vi "Initialize Diagnostics Main.vi"(8 "error in (no error)":errorcluster, 10 "This VI":refnum<vi>, 11 "Parameters":T1={"Properties"={"Name"="", "CAN"={"Database File"=path "", "CAN Interface"=enum."CAN0", "Baud Rate"=0, "Diagnostic Protocol"=enum."GMLAN", "Transport Protocol"=enum."ISO TP - Normal Mode", "Transmit ID"=0, "Receive ID"=0, "Transmit Extension"=0, "Receive Extension"=0, "Receive UUDT ID"=0, "Enable Stream"=TRUE, "VW TP Channel ID"=0, "Security"={"Source DLL Path"=path "", "Security Level"=1, "Target DLL Path"=path ""}, "Fill Frame"=FALSE, "Fill Byte"=255, "Termination"=FALSE}, "FPGA Settings"={"RT Bitfile Path"=path "", "RIO Device"=0, "Enable"=FALSE}, "PIDs"=[], "PID Lookup"=variant, "CPIDs"=[], "CPID Lookup"=variant, "DIDs"=[], "DID Lookup"=variant, "DPIDs"=[], "DPID Lookup"=variant, "DTC descriptor"={"DTC Byte Length"=2, "Status Byte Length"=1, "Add Data Byte Length"=1, "Byte Order"=enum."Motorola"}, "Routine.Start.Cmd Lookup"=variant, "Routine.Status.Cmd Lookup"=variant, "Routine.Stop.Cmd Lookup"=variant, "IO.Cmd Lookup"=variant, "IO.Resp Lookup"=variant, "Routine.Start.Resp Lookup"=variant, "Routine.Status.Resp Lookup"=variant, "Routine.Stop.Resp Lookup"=variant, "Memory.Write Lookup"=variant, "Memory.Read Lookup"=variant}, "ChanRefs"={"ToVS.PIDs"={"Name"="", "Write to VS Engine FIFO"=refnum, "Pairs"={"Refs"=[], "Values"=[]}}, "ToVS.DIDs"={"Name"="", "Write to VS Engine FIFO"=refnum, "Pairs"={"Refs"=[], "Values"=[]}}, "ToVS.DTCs"={"Name"="", "Write to VS Engine FIFO"=refnum, "Pairs"={"Refs"=[], "Values"=[]}}, "ToVS.DTCCount"={"Name"="", "Write to VS Engine FIFO"=refnum, "Pairs"={"Refs"=[], "Values"=[]}}, "ToVS.Status"={"Name"="", "Write to VS Engine FIFO"=refnum, "Pairs"={"Refs"=[], "Values"=[]}}, "FromVS.CPIDs"={"Name"="", "Read from VS Engine FIFO"=refnum, "Pairs"={"Refs"=[], "Values"=[]}}, "Cmds"={"Name"="", "Write to VS Engine FIFO"=refnum, "Read from VS Engine FIFO"=refnum, "Pairs"={"Chan Refs"=[], "Prev. Values"=[]}}, "ToVS.Routine.Start"={"Name"="", "Write to VS Engine FIFO"=refnum, "Pairs"={"Refs"=[], "Values"=[]}}, "FromVS.Routine.Start"={"Name"="", "Read from VS Engine FIFO"=refnum, "Pairs"={"Refs"=[], "Values"=[]}}, "ToVS.Routine.Stop"={"Name"="", "Write to VS Engine FIFO"=refnum, "Pairs"={"Refs"=[], "Values"=[]}}, "FromVS.Routine.Stop"={"Name"="", "Read from VS Engine FIFO"=refnum, "Pairs"={"Refs"=[], "Values"=[]}}, "ToVS.Routine.Status"={"Name"="", "Write to VS Engine FIFO"=refnum, "Pairs"={"Refs"=[], "Values"=[]}}, "FromVS.Routine.Status"={"Name"="", "Read from VS Engine FIFO"=refnum, "Pairs"={"Refs"=[], "Values"=[]}}, "FromVS.IO.Cmd"={"Name"="", "Read from VS Engine FIFO"=refnum, "Pairs"={"Refs"=[], "Values"=[]}}, "ToVS.IO.Resp"={"Name"="", "Write to VS Engine FIFO"=refnum, "Pairs"={"Refs"=[], "Values"=[]}}, "FromVS.WriteMemory"={"Name"="", "Read from VS Engine FIFO"=refnum, "Pairs"={"Refs"=[], "Values"=[]}}, "ToVS.ReadMemory"={"Name"="", "Write to VS Engine FIFO"=refnum, "Pairs"={"Refs"=[], "Values"=[]}}}} {"ChanRefs"."ToVS.ReadMemory"."Pairs"."Refs" format="%.0x"; "ChanRefs"."FromVS.WriteMemory"."Pairs"."Refs"."Data Reference" format="%.0x"; "ChanRefs"."ToVS.IO.Resp"."Pairs"."Refs" format="%.0x"; "ChanRefs"."FromVS.IO.Cmd"."Pairs"."Refs"."Data Reference" format="%.0x"; "ChanRefs"."FromVS.Routine.Status"."Pairs"."Refs"."Data Reference" format="%.0x"; "ChanRefs"."ToVS.Routine.Status"."Pairs"."Refs" format="%.0x"; "ChanRefs"."FromVS.Routine.Stop"."Pairs"."Refs"."Data Reference" format="%.0x"; "ChanRefs"."ToVS.Routine.Stop"."Pairs"."Refs" format="%.0x"; "ChanRefs"."FromVS.Routine.Start"."Pairs"."Refs"."Data Reference" format="%.0x"; "ChanRefs"."ToVS.Routine.Start"."Pairs"."Refs" format="%.0x"; "ChanRefs"."Cmds"."Pairs"."Chan Refs" format="%.0x"; "ChanRefs"."FromVS.CPIDs"."Pairs"."Refs"."Data Reference" format="%.0x"; "ChanRefs"."ToVS.Status"."Pairs"."Refs" format="%.0x"; "ChanRefs"."ToVS.DTCCount"."Pairs"."Refs" format="%.0x"; "ChanRefs"."ToVS.DTCs"."Pairs"."Refs" format="%.0x"; "ChanRefs"."ToVS.PIDs"."Pairs"."Refs" format="%.0x"; "ChanRefs"."ToVS.DIDs"."Pairs"."Refs" format="%.0x"; "Properties"."CPIDs"."Signals"."Byte Order" items=["Little Endian", "Big Endian"]; "Properties"."CPIDs"."Signals"."Data Type" items=["Signed", "Unsigned", "IEEE Float"]; "Properties"."DIDs"."Signals"."Byte Order" items=["Little Endian", "Big Endian"]; "Properties"."DIDs"."Signals"."Data Type" items=["Signed", "Unsigned", "IEEE Float"]; "Properties"."CAN"."Fill Byte" format="%.0x"; "Properties"."CAN"."VW TP Channel ID" format="%.0x"; "Properties"."CAN"."Receive UUDT ID" format="%.0x"; "Properties"."CAN"."Receive Extension" format="%.0x"; "Properties"."CAN"."Transmit Extension" format="%.0x"; "Properties"."CAN"."Receive ID" format="%.0x"; "Properties"."CAN"."Transmit ID" format="%.0x"; "Properties"."PIDs"."Signals"."Byte Order" items=["Little Endian", "Big Endian"]; "Properties"."PIDs"."Signals"."Data Type" items=["Signed", "Unsigned", "IEEE Float"]}) -> (0 "error out":errorcluster {"code" min=0 max=0}, 3 "State Variables Out":T20={"TCP Refs"={"Connection List"=refnum, "listener ID"=refnum}, "Stop"=refnum, "Top VI"=refnum, "Parameters"={"Properties"={"Name"="", "CAN"={"Database File"=path "", "CAN Interface"=enum."CAN0", "Baud Rate"=0, "Diagnostic Protocol"=enum."GMLAN", "Transport Protocol"=enum."ISO TP - Normal Mode", "Transmit ID"=0, "Receive ID"=0, "Transmit Extension"=0, "Receive Extension"=0, "Receive UUDT ID"=0, "Enable Stream"=TRUE, "VW TP Channel ID"=0, "Security"={"Source DLL Path"=path "", "Security Level"=1, "Target DLL Path"=path ""}, "Fill Frame"=FALSE, "Fill Byte"=255, "Termination"=FALSE}, "FPGA Settings"={"RT Bitfile Path"=path "", "RIO Device"=0, "Enable"=FALSE}, "PIDs"=[], "PID Lookup"=variant, "CPIDs"=[], "CPID Lookup"=variant, "DIDs"=[], "DID Lookup"=variant, "DPIDs"=[], "DPID Lookup"=variant, "DTC descriptor"={"DTC Byte Length"=2, "Status Byte Length"=1, "Add Data Byte Length"=1, "Byte Order"=enum."Motorola"}, "Routine.Start.Cmd Lookup"=variant, "Routine.Status.Cmd Lookup"=variant, "Routine.Stop.Cmd Lookup"=variant, "IO.Cmd Lookup"=variant, "IO.Resp Lookup"=variant, "Routine.Start.Resp Lookup"=variant, "Routine.Status.Resp Lookup"=variant, "Routine.Stop.Resp Lookup"=variant, "Memory.Write Lookup"=variant, "Memory.Read Lookup"=variant}, "ChanRefs"={"ToVS.PIDs"={"Name"="", "Write to VS Engine FIFO"=refnum, "Pairs"={"Refs"=[], "Values"=[]}}, "ToVS.DIDs"={"Name"="", "Write to VS Engine FIFO"=refnum, "Pairs"={"Refs"=[], "Values"=[]}}, "ToVS.DTCs"={"Name"="", "Write to VS Engine FIFO"=refnum, "Pairs"={"Refs"=[], "Values"=[]}}, "ToVS.DTCCount"={"Name"="", "Write to VS Engine FIFO"=refnum, "Pairs"={"Refs"=[], "Values"=[]}}, "ToVS.Status"={"Name"="", "Write to VS Engine FIFO"=refnum, "Pairs"={"Refs"=[], "Values"=[]}}, "FromVS.CPIDs"={"Name"="", "Read from VS Engine FIFO"=refnum, "Pairs"={"Refs"=[], "Values"=[]}}, "Cmds"={"Name"="", "Write to VS Engine FIFO"=refnum, "Read from VS Engine FIFO"=refnum, "Pairs"={"Chan Refs"=[], "Prev. Values"=[]}}, "ToVS.Routine.Start"={"Name"="", "Write to VS Engine FIFO"=refnum, "Pairs"={"Refs"=[], "Values"=[]}}, "FromVS.Routine.Start"={"Name"="", "Read from VS Engine FIFO"=refnum, "Pairs"={"Refs"=[], "Values"=[]}}, "ToVS.Routine.Stop"={"Name"="", "Write to VS Engine FIFO"=refnum, "Pairs"={"Refs"=[], "Values"=[]}}, "FromVS.Routine.Stop"={"Name"="", "Read from VS Engine FIFO"=refnum, "Pairs"={"Refs"=[], "Values"=[]}}, "ToVS.Routine.Status"={"Name"="", "Write to VS Engine FIFO"=refnum, "Pairs"={"Refs"=[], "Values"=[]}}, "FromVS.Routine.Status"={"Name"="", "Read from VS Engine FIFO"=refnum, "Pairs"={"Refs"=[], "Values"=[]}}, "FromVS.IO.Cmd"={"Name"="", "Read from VS Engine FIFO"=refnum, "Pairs"={"Refs"=[], "Values"=[]}}, "ToVS.IO.Resp"={"Name"="", "Write to VS Engine FIFO"=refnum, "Pairs"={"Refs"=[], "Values"=[]}}, "FromVS.WriteMemory"={"Name"="", "Read from VS Engine FIFO"=refnum, "Pairs"={"Refs"=[], "Values"=[]}}, "ToVS.ReadMemory"={"Name"="", "Write to VS Engine FIFO"=refnum, "Pairs"={"Refs"=[], "Values"=[]}}}}, "ADCS Connection"={"Diag CAN Handle"=0, "Transport Protocol"=enum."ISO TP - Normal Mode", "Receive Address Extension"=0, "Transmit Address Extension"=0, "Receive CAN Id"=0, "Transmit CAN Id"=0, "Diag CAN Queue"=refnum, "Log Frames ?"=FALSE, "My TP Address"=0, "Other TP Address"=0, "T1"=0, "T2"=0, "T3"=0, "T4"=0, "Tx SN"=0, "Block Size"=0, "Rx SN"=0, "VW TP Initialized?"=FALSE, "Tx block no"=0, "baud rate"=0, "Interface"="", "Channel Diag CAN Handle"=0, "UDP Connection ID"=refnum, "TCP Connection ID"=refnum, "Target IP Addr"=0, "Source Address"=0, "Target Address"=0, "Send Header NACK?"=FALSE, "DLL Handle"=0, "NAD"=0, "Time Stamp read first"=0.0, "Time Stamp read last"=0.0, "Time Stamp write first"=0.0, "Time Stamp write last"=0.0, "Time Stamp write"=0.0, "Time Stamp read"=0.0}, "XNET References"={"Database"="", "GMLAN DPID Session"="", "Cluster"=""}, "BufferedCmds"=refnum, "XNETEngine (GMLAN)"=refnum} {"Parameters"."ChanRefs"."ToVS.ReadMemory"."Pairs"."Refs" format="%.0x"; "Parameters"."ChanRefs"."ToVS.IO.Resp"."Pairs"."Refs" format="%.0x"; "Parameters"."ChanRefs"."ToVS.Routine.Status"."Pairs"."Refs" format="%.0x"; "Parameters"."ChanRefs"."ToVS.Routine.Stop"."Pairs"."Refs" format="%.0x"; "Parameters"."ChanRefs"."ToVS.Routine.Start"."Pairs"."Refs" format="%.0x"; "Parameters"."ChanRefs"."Cmds"."Pairs"."Chan Refs" format="%.0x"; "Parameters"."ChanRefs"."ToVS.Status"."Pairs"."Refs" format="%.0x"; "Parameters"."ChanRefs"."ToVS.DTCCount"."Pairs"."Refs" format="%.0x"; "Parameters"."ChanRefs"."ToVS.DTCs"."Pairs"."Refs" format="%.0x"; "Parameters"."ChanRefs"."ToVS.PIDs"."Pairs"."Refs" format="%.0x"; "Parameters"."ChanRefs"."ToVS.DIDs"."Pairs"."Refs" format="%.0x"; "Parameters"."Properties"."CPIDs"."Signals"."Byte Order" items=["Little Endian", "Big Endian"]; "Parameters"."Properties"."CPIDs"."Signals"."Data Type" items=["Signed", "Unsigned", "IEEE Float"]; "Parameters"."Properties"."DIDs"."Signals"."Byte Order" items=["Little Endian", "Big Endian"]; "Parameters"."Properties"."DIDs"."Signals"."Data Type" items=["Signed", "Unsigned", "IEEE Float"]; "Parameters"."Properties"."CAN"."Fill Byte" format="%.0x"; "Parameters"."Properties"."CAN"."VW TP Channel ID" format="%.0x"; "Parameters"."Properties"."CAN"."Receive UUDT ID" format="%.0x"; "Parameters"."Properties"."CAN"."Receive Extension" format="%.0x"; "Parameters"."Properties"."CAN"."Transmit Extension" format="%.0x"; "Parameters"."Properties"."CAN"."Receive ID" format="%.0x"; "Parameters"."Properties"."CAN"."Transmit ID" format="%.0x"; "Parameters"."Properties"."PIDs"."Signals"."Byte Order" items=["Little Endian", "Big Endian"]; "Parameters"."Properties"."PIDs"."Signals"."Data Type" items=["Signed", "Unsigned", "IEEE Float"]})   [LabVIEW 2015, in "Diagnostics Addon Engine.lvlib"]
uses:
  Diagnostics Addon Engine.lvlib
  Types/State Variables.ctl
  Types/TCP Refs.ctl
  STM/STM Lookup Table Ref.ctl
  Stop FG/Stop Global Ref.ctl
  Types/Main Configuration.ctl
  Shared/Types/Section Properties.ctl
  Shared/Types/CAN Configuration.ctl
  Shared/Types/CAN Interface.ctl
  Shared/Types/Diagnostic Protocols.ctl
  Shared/Types/Transport Protocols.ctl
  Shared/Types/Security.ctl
  Shared/Types/FPGA Bitfile Settings.ctl
  Shared/Types/Frame Parameters.ctl
  Shared/Types/Signal Parameters.ctl
  Shared/Types/DPID Parameters.ctl
  Shared/Types/DPID Periodic Rate.ctl
  <vilib>/Automotive Diagnostic Command Set/Diagnostic Protocols.llb/DTC Descriptor.ctl
  Types/VS Data Channels.ctl
  Inline Async API/Controls/Write To VS Engine.ctl
  <vilib>/NI Veristand/Custom Device API/Data Reference.ctl
  Inline Async API/Controls/Read From VS Engine.ctl
  <vilib>/NI Veristand/Custom Device API/Block Data Reference.ctl
  Inline Async API/Controls/ReadWrite Data.ctl
  <vilib>/Automotive Diagnostic Command Set/Diagnostic Transport.llb/Diag Reference.ctl
  <vilib>/Automotive Diagnostic Command Set/Diagnostic Transport.llb/Transport Protocol Selector.ctl
  <vilib>/Automotive Diagnostic Command Set/Diagnostic Transport.llb/Diag CAN Frame Log.ctl
  Types/XNET References.ctl
  <vilib>/NI/AMC/Message Queue.ctl
  <vilib>/NI/AMC/Message.ctl
  <vilib>/NI/Tools/Keyed Array/KeyedArray.ctl
  Shared/SubVIs/GUID Lookup.vi
  STM/RQST Comm Lookup Table_Initialize.vi
  Stop FG/Stop FG.lvlib
  Shared/Diagnostics Addon Shared.lvlib
  <vilib>/NI Veristand/Custom Device API/Custom Device API.lvlib
  <vilib>/NI/AMC/AMC.lvlib
  <vilib>/NI/Tools/Keyed Array/Tools_KeyedArray.lvlib
  <vilib>/addons/Automotive Diagnostic Command Set/NI_Automotive Diagnostic Command Set.lvlib
  Inline Async API/Inline Async API.lvlib
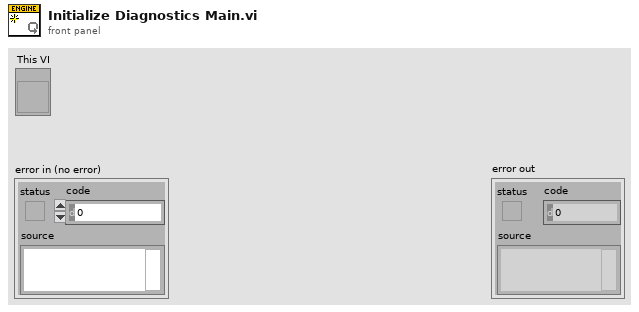
[diagram p1: front panel]
types:
  T1 = typedef "Diagnostics Addon Engine.lvlib/Main Configuration.ctl" = cluster{"Properties":T2, "ChanRefs":T14}
  T2 = typedef "Diagnostics Addon Shared.lvlib/Section Properties.ctl" = cluster{"Name":string, "CAN":T3, "FPGA Settings":T8, "PIDs":T9[], "PID Lookup":variant, "CPIDs":T9[], "CPID Lookup":variant, "DIDs":T9[], "DID Lookup":variant, "DPIDs":T11[], "DPID Lookup":variant, "DTC descriptor":T13, "Routine.Start.Cmd Lookup":variant, "Routine.Status.Cmd Lookup":variant, "Routine.Stop.Cmd Lookup":variant, "IO.Cmd Lookup":variant, "IO.Resp Lookup":variant, "Routine.Start.Resp Lookup":variant, "Routine.Status.Resp Lookup":variant, "Routine.Stop.Resp Lookup":variant, "Memory.Write Lookup":variant, "Memory.Read Lookup":variant}
  T3 = typedef "Diagnostics Addon Shared.lvlib/CAN Configuration.ctl" = cluster{"Database File":path, "CAN Interface":T4, "Baud Rate":u32, "Diagnostic Protocol":T5, "Transport Protocol":T6, "Transmit ID":u32, "Receive ID":u32, "Transmit Extension":u8, "Receive Extension":u8, "Receive UUDT ID":u32, "Enable Stream":bool, "VW TP Channel ID":u32, "Security":T7, "Fill Frame":bool, "Fill Byte":u8, "Termination":bool}
  T4 = typedef "Diagnostics Addon Shared.lvlib/CAN Interface.ctl" = enum16{"CAN0", "CAN1", "CAN2", "CAN3", "CAN4", "CAN5", "CAN6", "CAN7", "CAN8", "CAN9", "CAN10", "CAN11", "CAN12", "CAN13", "CAN14", "CAN15", "CAN16", "CAN17", "CAN18", "CAN19", "CAN20", "CAN21", "CAN22", "CAN23", "CAN24", "CAN25", "CAN26", "CAN27", "CAN28", "CAN29", "CAN30", "CAN31", "CAN32", "CAN33", "CAN34", "CAN35", "CAN36", "CAN37", "CAN38", "CAN39", "CAN40", "CAN41", "CAN42", "CAN43", "CAN44", "CAN45", "CAN46", "CAN47", "CAN48", "CAN49", "CAN50", "CAN51", "CAN52", "CAN53", "CAN54", "CAN55", "CAN56", "CAN57", "CAN58", "CAN59", "CAN60", "CAN61", "CAN62", "CAN63", "CAN 256 (Virtual)", "CAN 257 (Virtual)"}
  T5 = typedef "Diagnostics Addon Shared.lvlib/Diagnostic Protocols.ctl" = enum16{"GMLAN", "KWP-2000", "UDS"}
  T6 = typedef "Diagnostics Addon Shared.lvlib/Transport Protocols.ctl" = enum16{"ISO TP - Normal Mode", "ISO TP - Mixed Mode", "VW TP 2.0", "Diagnostics on IP"}
  T7 = typedef "Diagnostics Addon Shared.lvlib/Security.ctl" = cluster{"Source DLL Path":path, "Security Level":u8, "Target DLL Path":path}
  T8 = typedef "Diagnostics Addon Shared.lvlib/FPGA Bitfile Settings.ctl" = cluster{"RT Bitfile Path":path, "RIO Device":u16, "Enable":bool}
  T9 = typedef "Diagnostics Addon Shared.lvlib/Frame Parameters.ctl" = cluster{"Name":string, "Description":string, "ID":u16, "Signals":T10[]}
  T10 = typedef "Diagnostics Addon Shared.lvlib/Signal Parameters.ctl" = cluster{"Start Bit":u8, "Length":u8, "Scaling Factor":dbl, "Scaling Offset":dbl, "Minimum":dbl, "Maximum":dbl, "Data Type":u32, "Byte Order":u32, "Default Value":dbl, "Name":string, "Units":string, "Description":string}
  T11 = typedef "Diagnostics Addon Shared.lvlib/DPID Parameters.ctl" = cluster{"DPID ID":u8, "Speed":T12, "PIDs":u16[]}
  T12 = typedef "Diagnostics Addon Shared.lvlib/DPID Periodic Rate.ctl" = enum16{"Slow", "Medium", "Fast"}
  T13 = typedef "Diagnostics Addon Shared.lvlib/DTC Descriptor.ctl" = cluster{"DTC Byte Length":i32, "Status Byte Length":i32, "Add Data Byte Length":i32, "Byte Order":enum16{"Motorola", "Intel"}}
  T14 = typedef "Diagnostics Addon Engine.lvlib/VS Data Channels.ctl" = cluster{"ToVS.PIDs":T15, "ToVS.DIDs":T15, "ToVS.DTCs":T15, "ToVS.DTCCount":T15, "ToVS.Status":T15, "FromVS.CPIDs":T17, "Cmds":T19, "ToVS.Routine.Start":T15, "FromVS.Routine.Start":T17, "ToVS.Routine.Stop":T15, "FromVS.Routine.Stop":T17, "ToVS.Routine.Status":T15, "FromVS.Routine.Status":T17, "FromVS.IO.Cmd":T17, "ToVS.IO.Resp":T15, "FromVS.WriteMemory":T17, "ToVS.ReadMemory":T15}
  T15 = typedef "Diagnostics Addon Engine.lvlib/Inline Async API.lvlib/Write To VS Engine.ctl" = cluster{"Name":string, "Write to VS Engine FIFO":refnum<k33>, "Pairs":cluster{"Refs":T16[], "Values":dbl[]}}
  T16 = typedef "Custom Device API.lvlib/Data Reference.ctl" = i32
  T17 = typedef "Diagnostics Addon Engine.lvlib/Inline Async API.lvlib/Read From VS Engine.ctl" = cluster{"Name":string, "Read from VS Engine FIFO":refnum<k33>, "Pairs":cluster{"Refs":T18[], "Values":dbl[]}}
  T18 = typedef "Custom Device API.lvlib/Block Data Reference.ctl" = cluster{"Data Reference":T16, "Offset":u64, "Length":u64}
  T19 = typedef "Diagnostics Addon Engine.lvlib/Inline Async API.lvlib/ReadWrite Data.ctl" = cluster{"Name":string, "Write to VS Engine FIFO":refnum<k33>, "Read from VS Engine FIFO":refnum<k33>, "Pairs":cluster{"Chan Refs":T16[], "Prev. Values":dbl[]}}
  T20 = typedef "Diagnostics Addon Engine.lvlib/State Variables.ctl" = cluster{"TCP Refs":T21, "Stop":T23, "Top VI":refnum<vi>, "Parameters":T1, "ADCS Connection":T24, "XNET References":T26, "BufferedCmds":T27, "XNETEngine (GMLAN)":T27}
  T21 = typedef "Diagnostics Addon Engine.lvlib/TCP Refs.ctl" = cluster{"Connection List":T22, "listener ID":refnum<k5>}
  T22 = typedef "Diagnostics Addon Engine.lvlib/STM Lookup Table Ref.ctl" = refnum<vi>
  T23 = typedef "Diagnostics Addon Engine.lvlib/Stop FG.lvlib/Stop Global Ref.ctl" = refnum<vi>
  T24 = typedef "NI_Automotive Diagnostic Command Set.lvlib/Diag Reference.ctl" = cluster{"Diag CAN Handle":u32, "Transport Protocol":T25, "Receive Address Extension":u8, "Transmit Address Extension":u8, "Receive CAN Id":u32, "Transmit CAN Id":u32, "Diag CAN Queue":refnum<queue>, "Log Frames ?":bool, "My TP Address":u8, "Other TP Address":u8, "T1":u16, "T2":u16, "T3":u16, "T4":u16, "Tx SN":u8, "Block Size":u8, "Rx SN":u8, "VW TP Initialized?":bool, "Tx block no":u8, "baud rate":u32, "Interface":string, "Channel Diag CAN Handle":u32, "UDP Connection ID":refnum<k16>, "TCP Connection ID":refnum<k5>, "Target IP Addr":u32, "Source Address":u16, "Target Address":u16, "Send Header NACK?":bool, "DLL Handle":u32, "NAD":u8, "Time Stamp read first":dbl, "Time Stamp read last":dbl, "Time Stamp write first":dbl, "Time Stamp write last":dbl, "Time Stamp write":dbl, "Time Stamp read":dbl}
  T25 = typedef "NI_Automotive Diagnostic Command Set.lvlib/Transport Protocol Selector.ctl" = enum16{"ISO TP - Normal Mode", "ISO TP - Mixed Mode", "VW TP 2.0", "Diagnostics on IP", "ISO TP LIN"}
  T26 = typedef "Diagnostics Addon Engine.lvlib/XNET References.ctl" = cluster{"Database":refnum<k21>, "GMLAN DPID Session":refnum<k21>, "Cluster":refnum<k21>}
  T27 = typedef "AMC.lvlib/Message Queue.ctl" = refnum<queue>
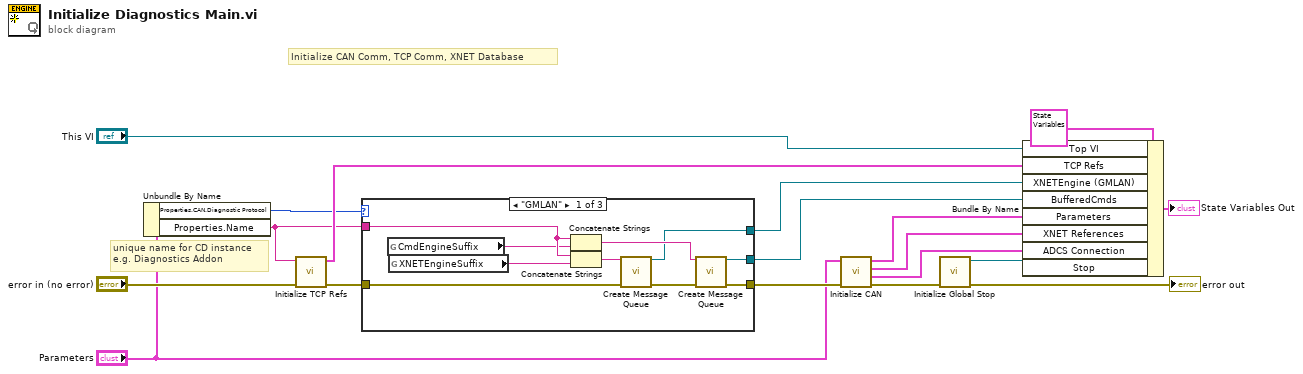
[diagram p0: block diagram]
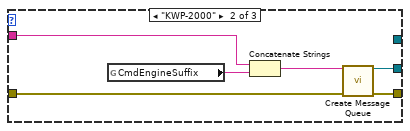
[diagram p2: hidden frame]
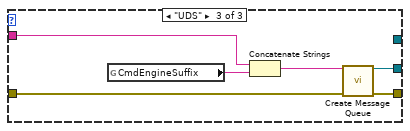
[diagram p3: hidden frame]
diagram:
  # "unique name for CD instance\ne.g. Diagnostics Addon"
  # "Initialize CAN Comm, TCP Comm, XNET Database"
  n1 = Unbundle By Name("Parameters") -> ("Properties.CAN.Diagnostic Protocol"=w9:T5, "Properties.Name"=w10:string)
  n2 = call "Initialize TCP Refs.vi"("error in (no error)"="error in (no error)", "Name"=w10) -> ("error out"=w8:errorcluster, "TCP Refs"=w15:T21)  [unwired: 8 in]
  n3 = case shown="\"GMLAN\"" w9 {
    tunnel: w10 -> [w23 w31 w37]
    tunnel: [w24 w33 w39] -> w7
    tunnel: w8 -> [w25 w32 w38]
    tunnel: [w22 w30 w36] -> w5
    tunnel: [w21 _ _] -> w6
    frame "GMLAN" {
      n4 = global read "GUID Lookup.vi" "CmdEngineSuffix"() -> (w19:string)
      n5 = global read "GUID Lookup.vi" "XNETEngineSuffix"() -> (w20:string)
      n6 = Concatenate Strings(w23, w19) -> (w26:string)
      n7 = Concatenate Strings(w23, w20) -> (w27:string)
      n8 = call <vilib>:"Create Message Queue.vi"("message queue name"=w27, "error in"=w25) -> ("message queue out"=w21:T27, "error out"=w28:errorcluster)  [unwired: 12 in]
      n9 = call <vilib>:"Create Message Queue.vi"("message queue name"=w26, "error in"=w28) -> ("message queue out"=w22:T27, "error out"=w24:errorcluster)  [unwired: 12 in]
    }
    frame "KWP-2000" {
      n10 = global read "GUID Lookup.vi" "CmdEngineSuffix"() -> (w29:string)
      n11 = Concatenate Strings(w31, w29) -> (w34:string)
      n12 = call <vilib>:"Create Message Queue.vi"("message queue name"=w34, "error in"=w32) -> ("message queue out"=w30:T27, "error out"=w33:errorcluster)  [unwired: 12 in]
    }
    frame "UDS" {
      n13 = global read "GUID Lookup.vi" "CmdEngineSuffix"() -> (w35:string)
      n14 = Concatenate Strings(w37, w35) -> (w40:string)
      n15 = call <vilib>:"Create Message Queue.vi"("message queue name"=w40, "error in"=w38) -> ("message queue out"=w36:T27, "error out"=w39:errorcluster)  [unwired: 12 in]
    }
  }
  n16 = call "Initialize CAN.vi"("error in (no error)"=w7, "Parameters"="Parameters") -> ("error out"=w11:errorcluster, "ADCS Connection"=w4:T24, "XNET References"=w2:T26, "Parameters"=w3:T1)  [unwired: 6 in]
  n17 = call "Initialize Global Stop.vi"("error in (no error)"=w11) -> ("error out"=→"error out":errorcluster, "vi reference"=w13:T23)  [unwired: 9 in]
  n18 = Bundle By Name(cluster=T20 {"TCP Refs"={"Connection List"=refnum, "listener ID"=refnum}, "Stop"=refnum, "Top VI"=refnum, "Parameters"={"Properties"={"Name"="", "CAN"={"Database File"=path "", "CAN Interface"=enum."CAN0", "Baud Rate"=0, "Diagnostic Protocol"=enum."GMLAN", "Transport Protocol"=enum."ISO TP - Normal Mode", "Transmit ID"=0, "Receive ID"=0, "Transmit Extension"=0, "Receive Extension"=0, "Receive UUDT ID"=0, "Enable Stream"=FALSE, "VW TP Channel ID"=0, "Security"={"Source DLL Path"=path "", "Security Level"=1, "Target DLL Path"=path ""}, "Fill Frame"=FALSE, "Fill Byte"=255, "Termination"=FALSE}, "FPGA Settings"={"RT Bitfile Path"=path "", "RIO Device"=0, "Enable"=FALSE}, "PIDs"=[], "PID Lookup"=variant, "CPIDs"=[], "CPID Lookup"=variant, "DIDs"=[], "DID Lookup"=variant, "DPIDs"=[], "DPID Lookup"=variant, "DTC descriptor"={"DTC Byte Length"=0, "Status Byte Length"=0, "Add Data Byte Length"=0, "Byte Order"=enum."Motorola"}, "Routine.Start.Cmd Lookup"=variant, "Routine.Status.Cmd Lookup"=variant, "Routine.Stop.Cmd Lookup"=variant, "IO.Cmd Lookup"=variant, "IO.Resp Lookup"=variant, "Routine.Start.Resp Lookup"=variant, "Routine.Status.Resp Lookup"=variant, "Routine.Stop.Resp Lookup"=variant, "Memory.Write Lookup"=variant, "Memory.Read Lookup"=variant}, "ChanRefs"={"ToVS.PIDs"={"Name"="", "Write to VS Engine FIFO"=refnum, "Pairs"={"Refs"=[], "Values"=[]}}, "ToVS.DIDs"={"Name"="", "Write to VS Engine FIFO"=refnum, "Pairs"={"Refs"=[], "Values"=[]}}, "ToVS.DTCs"={"Name"="", "Write to VS Engine FIFO"=refnum, "Pairs"={"Refs"=[], "Values"=[]}}, "ToVS.DTCCount"={"Name"="", "Write to VS Engine FIFO"=refnum, "Pairs"={"Refs"=[], "Values"=[]}}, "ToVS.Status"={"Name"="", "Write to VS Engine FIFO"=refnum, "Pairs"={"Refs"=[], "Values"=[]}}, "FromVS.CPIDs"={"Name"="", "Read from VS Engine FIFO"=refnum, "Pairs"={"Refs"=[], "Values"=[]}}, "Cmds"={"Name"="", "Write to VS Engine FIFO"=refnum, "Read from VS Engine FIFO"=refnum, "Pairs"={"Chan Refs"=[], "Prev. Values"=[]}}, "ToVS.Routine.Start"={"Name"="", "Write to VS Engine FIFO"=refnum, "Pairs"={"Refs"=[], "Values"=[]}}, "FromVS.Routine.Start"={"Name"="", "Read from VS Engine FIFO"=refnum, "Pairs"={"Refs"=[], "Values"=[]}}, "ToVS.Routine.Stop"={"Name"="", "Write to VS Engine FIFO"=refnum, "Pairs"={"Refs"=[], "Values"=[]}}, "FromVS.Routine.Stop"={"Name"="", "Read from VS Engine FIFO"=refnum, "Pairs"={"Refs"=[], "Values"=[]}}, "ToVS.Routine.Status"={"Name"="", "Write to VS Engine FIFO"=refnum, "Pairs"={"Refs"=[], "Values"=[]}}, "FromVS.Routine.Status"={"Name"="", "Read from VS Engine FIFO"=refnum, "Pairs"={"Refs"=[], "Values"=[]}}, "FromVS.IO.Cmd"={"Name"="", "Read from VS Engine FIFO"=refnum, "Pairs"={"Refs"=[], "Values"=[]}}, "ToVS.IO.Resp"={"Name"="", "Write to VS Engine FIFO"=refnum, "Pairs"={"Refs"=[], "Values"=[]}}, "FromVS.WriteMemory"={"Name"="", "Read from VS Engine FIFO"=refnum, "Pairs"={"Refs"=[], "Values"=[]}}, "ToVS.ReadMemory"={"Name"="", "Write to VS Engine FIFO"=refnum, "Pairs"={"Refs"=[], "Values"=[]}}}}, "ADCS Connection"={"Diag CAN Handle"=0, "Transport Protocol"=enum."ISO TP - Normal Mode", "Receive Address Extension"=0, "Transmit Address Extension"=0, "Receive CAN Id"=0, "Transmit CAN Id"=0, "Diag CAN Queue"=refnum, "Log Frames ?"=FALSE, "My TP Address"=0, "Other TP Address"=0, "T1"=0, "T2"=0, "T3"=0, "T4"=0, "Tx SN"=0, "Block Size"=0, "Rx SN"=0, "VW TP Initialized?"=FALSE, "Tx block no"=0, "baud rate"=0, "Interface"="", "Channel Diag CAN Handle"=0, "UDP Connection ID"=refnum, "TCP Connection ID"=refnum, "Target IP Addr"=0, "Source Address"=0, "Target Address"=0, "Send Header NACK?"=FALSE, "DLL Handle"=0, "NAD"=0, "Time Stamp read first"=0.0, "Time Stamp read last"=0.0, "Time Stamp write first"=0.0, "Time Stamp write last"=0.0, "Time Stamp write"=0.0, "Time Stamp read"=0.0}, "XNET References"={"Database"="", "GMLAN DPID Session"="", "Cluster"=""}, "BufferedCmds"=refnum, "XNETEngine (GMLAN)"=refnum} ("State Variables"), "Top VI"="This VI", "TCP Refs"=w15, "XNETEngine (GMLAN)"=w6, "BufferedCmds"=w5, "Parameters"=w3, "XNET References"=w2, "ADCS Connection"=w4, "Stop"=w13) -> (→"State Variables Out":T20)
